vi "Serialize - Text.vi"(8 "error in":errorcluster, 11 "CRDS Cell Data in":refnum<class "CRDS Cell Data.lvclass">) -> (0 "error out":errorcluster, 2 "Serialized Text":string, 3 "CRDS Cell Data out":refnum<class "CRDS Cell Data.lvclass">)   [LabVIEW 2016, in "CRDS Lib.lvlib" / "CRDS Cell Data.lvclass"]
uses:
  CRDS Cell Data.lvclass
  CRDS Cell Data.lvclass/CRDS Cell Data.ctl
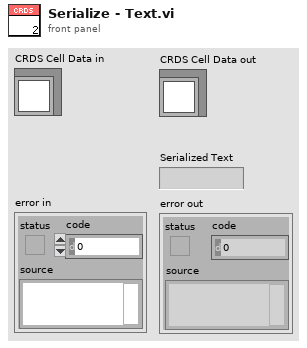
[diagram p1: front panel]
types:
  T1 = typedef "CRDS Lib.lvlib/CRDS Cell Data.lvclass/extParam Ctl.ctl" = cluster{"Tau":sgl, "Tau0cor":sgl, "ext":sgl, "extCorr":sgl, "stdevTau":sgl, "eTau":sgl, "taucorr":sgl, "Tau0":sgl, "max":sgl}
  T2 = typedef "CRDS Lib.lvlib/CRDS Cell Data.lvclass/hkParam Ctl.ctl" = cluster{"rhDilFac":sgl, "Q":sgl, "Tmean":sgl, "extDilFac":sgl, "rhCell":sgl, "P":sgl, "T":sgl}
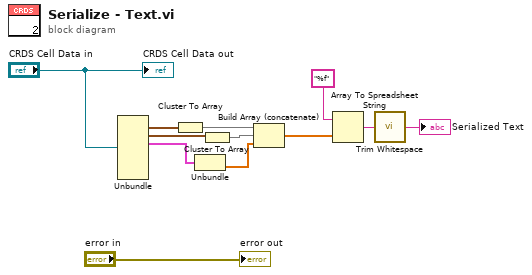
[diagram p0: block diagram]
diagram:
  n1 = Unbundle("CRDS Cell Data in") -> (w10:T1, w9:T2, w2:cluster{"ChunkSize":i32[], "StdDev":sgl[]})  [unwired: 5 out]
  n2 = Cluster To Array(cluster=w10) -> (array=w8:sgl[])
  n3 = Unbundle(w2) -> ("StdDev"=w1:sgl[])  [unwired: 1 out]
  n4 = Cluster To Array(cluster=w9) -> (array=w7:sgl[])
  n5 = Build Array (concatenate)(w8, w7, w1) -> (w6:sgl[])
  n6 = Array To Spreadsheet String(array=w6, 3:"%f" ("format string")) -> (spreadsheet string=w4:string)  [unwired: 1 in]
  n7 = call <vilib>:"Trim Whitespace.vi"("string"=w4) -> ("trimmed string"=→"Serialized Text":string)  [unwired: 1 in]
  "error out" <- "error in"
  "CRDS Cell Data out" <- "CRDS Cell Data in"
